vi "Parse LabVIEW Project File for Additional Installers.vi"(8 "error in (no error)":errorcluster, 10 "Build Specification Name (\"\" = first installer)":string, 11 "LabVIEW Project Path":path) -> (0 "error out":errorcluster, 3 "Additional Installers":T1[](array[typedef]))   [LabVIEW 2017, in "LabVIEW Installer Support.lvlib"]
doc: "Retrieves the list of additional installers from a LabVIEW project file."
uses:
  LabVIEW Installer Support.lvlib
  Additional Installer.ctl
  Installer Soft Dep.ctl
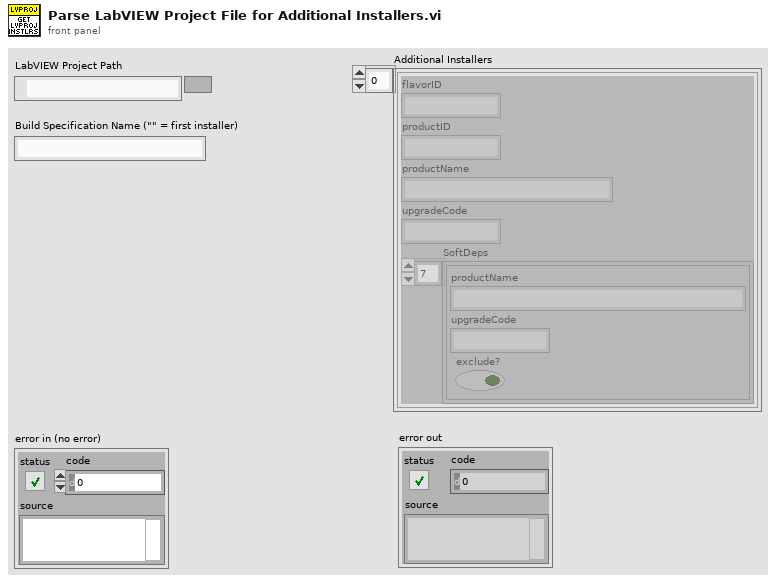
[diagram p1: front panel]
types:
  T1 = typedef "LabVIEW Installer Support.lvlib/Additional Installer.ctl" = cluster{"flavorID":string, "productID":string, "productName":string, "upgradeCode":string, "SoftDeps":T2[]}
  T2 = typedef "LabVIEW Installer Support.lvlib/Installer Soft Dep.ctl" = cluster{"productName":string, "upgradeCode":string, "exclude?":bool}
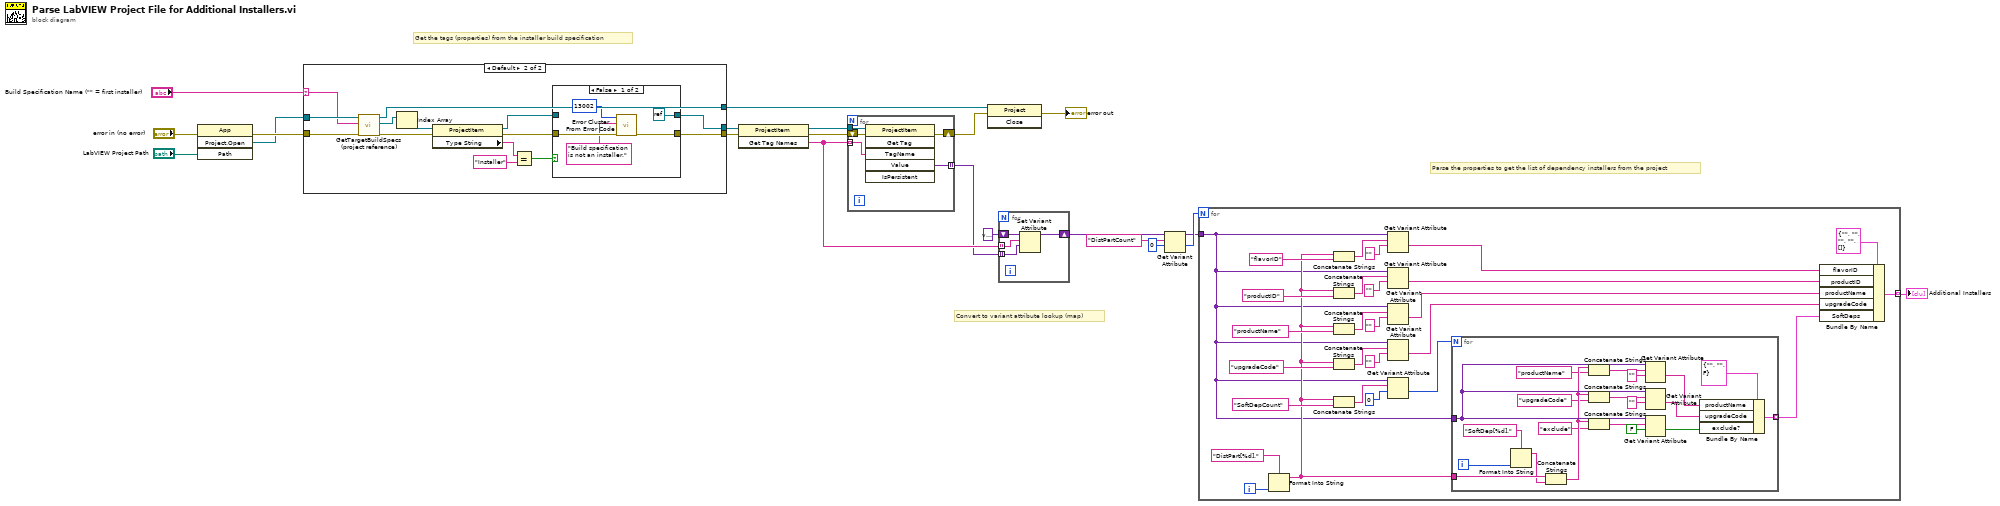
[diagram p0: block diagram]
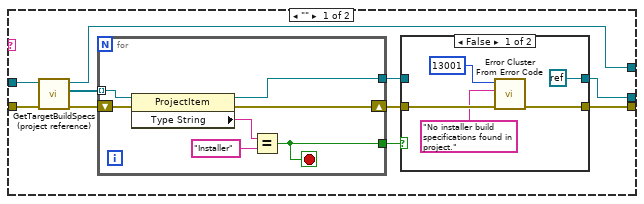
[diagram p2: hidden frame]
diagram:
  # "Parse the properties to get the list of dependency installers from the project"
  # "Convert to variant attribute lookup (map)"
  # "Get the tags (properties) from the installer build specification"
  n1 = invoke class="App" method="Project.Open"(error in="error in (no error)", "Path"="LabVIEW Project Path") -> (error out=w21:errorcluster, "Project:Open"=w20:refnum<vi>)  [unwired: 2 in, 2 out]
  n2 = case shown="Default" "Build Specification Name (\"\" = first installer)" {
    selector: "Build Specification Name (\"\" = first installer)" -> [_ w55]
    tunnel: w21 -> [w30 w58]
    tunnel: w20 -> [w31 w57]
    tunnel: [w25 w47] -> w19
    tunnel: [w23 w48] -> w18
    tunnel: [w27 w56] -> w17
    frame "" {
      n3 = call <vilib>:"GetTargetBuildSpecs (project reference).vi"("error in (no error)"=w30, "Project reference"=w31) -> ("error out"=w28:errorcluster, "buildspec refs"=w29:refnum<vi>[], "project ref"=w27:refnum<vi>)  [unwired: 7 in]
      n4 = for {
        tunnel: w29 -> [w44] mode=indexing
        shift-right: [w41] -> w24
        shift-left: w28 -> [w45]
        tunnel: [w42] -> w22
        tunnel: [w40] -> w26
        stop <- w40 stop-if-true
        n5 = property class="ProjectItem"(reference=w44, error in=w45) -> (reference out=w42:refnum<vi>, error out=w41:errorcluster, "Type String"=w43:string)
        n6 = Equal?(x=w43, y="Installer") -> (x = y?=w40:bool)
      }
      n7 = case shown="False" w26 {
        tunnel: [w34 w38] -> w25
        tunnel: w24 -> [w35 w38]
        tunnel: [refnum<k0> refnum w37] -> w23
        tunnel: w22 -> [_ w37]
        frame False {
          n8 = call <vilib>:"Error Cluster From Error Code.vi"("error in (no error)"=w35, "error message (\"\")"="No installer build specifications found in project.", "error code (0)"=13001) -> ("error out"=w34:errorcluster)  [unwired: 6 in]
        }
        frame True {
        }
      }
    }
    frame Default {
      n9 = call <vilib>:"GetTargetBuildSpecs (project reference).vi"("error in (no error)"=w58, "Name of build specification (if empty: get all)"=w55, "Project reference"=w57) -> ("error out"=w52:errorcluster, "buildspec refs"=w59:refnum<vi>[], "project ref"=w56:refnum<vi>)  [unwired: 6 in]
      n10 = Index Array(array=w59) -> (element=w51:refnum<vi>)  [unwired: 1 in]
      n11 = property class="ProjectItem"(reference=w51, error in=w52) -> (reference out=w49:refnum<vi>, error out=w50:errorcluster, "Type String"=w54:string)
      n12 = Equal?(x=w54, y="Installer") -> (x = y?=w46:bool)
      n13 = case shown="False" w46 {
        tunnel: [w62 w66] -> w47
        tunnel: w50 -> [w63 w66]
        tunnel: [refnum<k0> refnum w65] -> w48
        tunnel: w49 -> [_ w65]
        frame False {
          n14 = call <vilib>:"Error Cluster From Error Code.vi"("error in (no error)"=w63, "error message (\"\")"="Build specification is not an installer.", "error code (0)"=13002) -> ("error out"=w62:errorcluster)  [unwired: 6 in]
        }
        frame True {
        }
      }
    }
  }
  n15 = invoke class="ProjectItem" method="Get Tag Names"(reference=w18, error in=w19) -> (reference out=w15:refnum<vi>, error out=w16:errorcluster, "Get Tag Names"=w12:string[])  [unwired: 1 in]
  n16 = for {
    tunnel: w15 -> [w70]
    shift-right: [w69] -> w14
    shift-left: w16 -> [w71]
    tunnel: w12 -> [w68] mode=indexing
    tunnel: [w67] -> w11 mode=indexing
    n17 = invoke class="ProjectItem" method="Get Tag"(reference=w70, error in=w71, "TagName"=w68) -> (error out=w69:errorcluster, "Value"=w67:variant)  [unwired: 3 in, 4 out]
  }
  n18 = invoke class="Project" method="Close"(reference=w17, error in=w14) -> (error out=→"error out":errorcluster)  [unwired: 1 in, 2 out]
  n19 = for {
    shift-right: [w74] -> w10
    shift-left: variant -> [w75]
    tunnel: w12 -> [w73] mode=indexing
    tunnel: w11 -> [w72] mode=indexing
    n20 = Set Variant Attribute(Variant=w75, name=w73, value=w72) -> (Variant out=w74:variant)  [unwired: 1 in, 2 out]
  }
  n21 = Get Variant Attribute(Variant=w10, name="DistPartCount" ("element"), default value (empty Variant)=0) -> (duplicate Variant=w6:variant, value=w7:i32)  [unwired: 1 in, 2 out]
  n22 = for {
    N: w7 -> [_]
    tunnel: w6 -> [w78]
    tunnel: [w76] -> w5 mode=indexing
    i -> [w101]
    n23 = Format Into String(format string="DistPart[%d].", w101) -> (resulting string=w79:string)  [unwired: 2 in, 1 out]
    n24 = Concatenate Strings(w79, "flavorID" ("string")) -> (w97:string)
    n25 = Concatenate Strings(w79, "productID" ("string")) -> (w95:string)
    n26 = Concatenate Strings(w79, "productName" ("string")) -> (w90:string)
    n27 = Concatenate Strings(w79, "upgradeCode" ("string")) -> (w89:string)
    n28 = Concatenate Strings(w79, "SoftDepCount" ("string")) -> (w84:string)
    n29 = Get Variant Attribute(Variant=w78, name=w97, default value (empty Variant)="") -> (value=w96:string)  [unwired: 1 in, 3 out]
    n30 = Get Variant Attribute(Variant=w78, name=w95, default value (empty Variant)="") -> (value=w83:string)  [unwired: 1 in, 3 out]
    n31 = Get Variant Attribute(Variant=w78, name=w90, default value (empty Variant)="") -> (value=w82:string)  [unwired: 1 in, 3 out]
    n32 = Get Variant Attribute(Variant=w78, name=w89, default value (empty Variant)="") -> (value=w81:string)  [unwired: 1 in, 3 out]
    n33 = Get Variant Attribute(Variant=w78, name=w84, default value (empty Variant)=0) -> (value=w80:i32)  [unwired: 1 in, 3 out]
    n34 = for {
      N: w80 -> [_]
      tunnel: w79 -> [w120]
      tunnel: w78 -> [w113]
      tunnel: [w117] -> w77 mode=indexing
      i -> [w121]
      n35 = Format Into String(format string="SoftDep[%d].", w121) -> (resulting string=w119:string)  [unwired: 2 in, 1 out]
      n36 = Concatenate Strings(w120, w119) -> (w108:string)
      n37 = Concatenate Strings(w108, "productName" ("string")) -> (w109:string)
      n38 = Concatenate Strings(w108, "upgradeCode" ("string")) -> (w107:string)
      n39 = Concatenate Strings(w108, "exclude" ("string")) -> (w106:string)
      n40 = Get Variant Attribute(Variant=w113, name=w109, default value (empty Variant)="") -> (value=w115:string)  [unwired: 1 in, 3 out]
      n41 = Get Variant Attribute(Variant=w113, name=w107, default value (empty Variant)="") -> (value=w110:string)  [unwired: 1 in, 3 out]
      n42 = Get Variant Attribute(Variant=w113, name=w106, default value (empty Variant)=FALSE) -> (value=w111:bool)  [unwired: 1 in, 3 out]
      n43 = Bundle By Name(cluster=T2 {"productName"="", "upgradeCode"="", "exclude?"=FALSE} ("Cluster"), "productName"=w115, "upgradeCode"=w110, "exclude?"=w111) -> (w117:T2)
    }
    n44 = Bundle By Name(cluster=T1 {"flavorID"="", "productID"="", "productName"="", "upgradeCode"="", "SoftDeps"=[]}, "flavorID"=w96, "productID"=w83, "productName"=w82, "upgradeCode"=w81, "SoftDeps"=w77) -> (w76:T1)
  }
  "Additional Installers" <- w5
